vi "Determinant of a 2x2 Matrix.vi"() -> ()   [LabVIEW 2018]
panel:
  out "Determinant":dbl
  in  "2X2 Matrix":dbl[][](array[numeric])
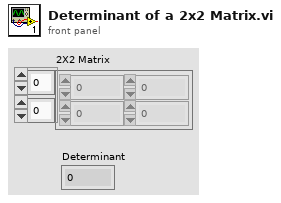
[diagram p1: front panel]
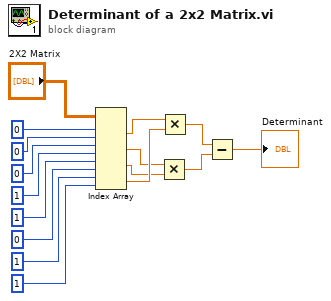
[diagram p0: block diagram]
diagram:
  n1 = Index Array(array="2X2 Matrix", index (row) #1=0, index (col) #1=0, index (row) #2=0, index (col) #2=1, index (row) #3=1, index (col) #3=0, index (row) #4=1, index (col) #4=1) -> (element #1=w4:dbl, element #2=w2:dbl, element #3=w1:dbl, element #4=w3:dbl)
  n2 = Multiply(x=w2, y=w1) -> (x*y=w6:dbl)
  n3 = Multiply(x=w4, y=w3) -> (x*y=w7:dbl)
  n4 = Subtract(x=w7, y=w6) -> (x-y=→"Determinant":dbl)
